vi "Netburner_cntl2.vi"() -> ()   [LabVIEW 2013]
panel:
  out "#  Bytes Read last":u32
  out "ADC last":string
  in  "Number of Cycles":i32=100
  out "ADC result":string
  out "#  Bytes Read":u32
  in  "ADC String  (Chan, #reads)":string="0 100"
  in  "2nd DAC String  (Chan, Volt)":string="1 -1."
  in  "1st DAC String  (Chan, Volt)":string="0 1"
  out "Error Out":errorcluster={"status"=FALSE, "code"=1073676294, "source"="VISA Read in Netburner_RD.vi->Netburner_cntl.vi"}
  in  "Error In (none)":errorcluster
  in  "COM Port #":refnum<visa-resource-name>="COM3"
  # "Netburner ADC/DAC Test Interface"
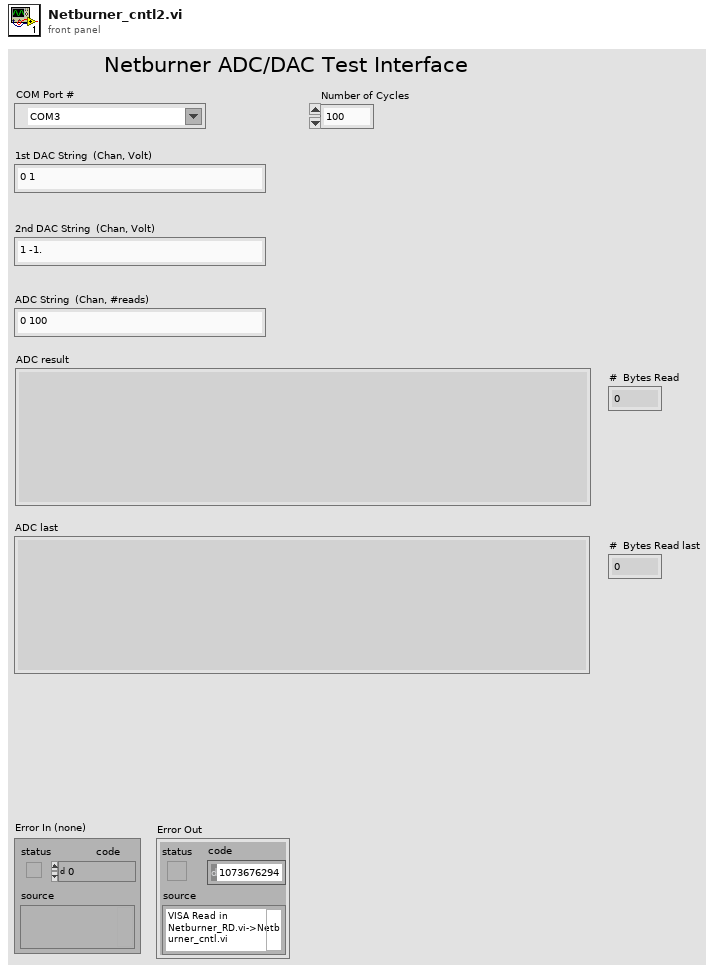
[diagram p1: front panel]
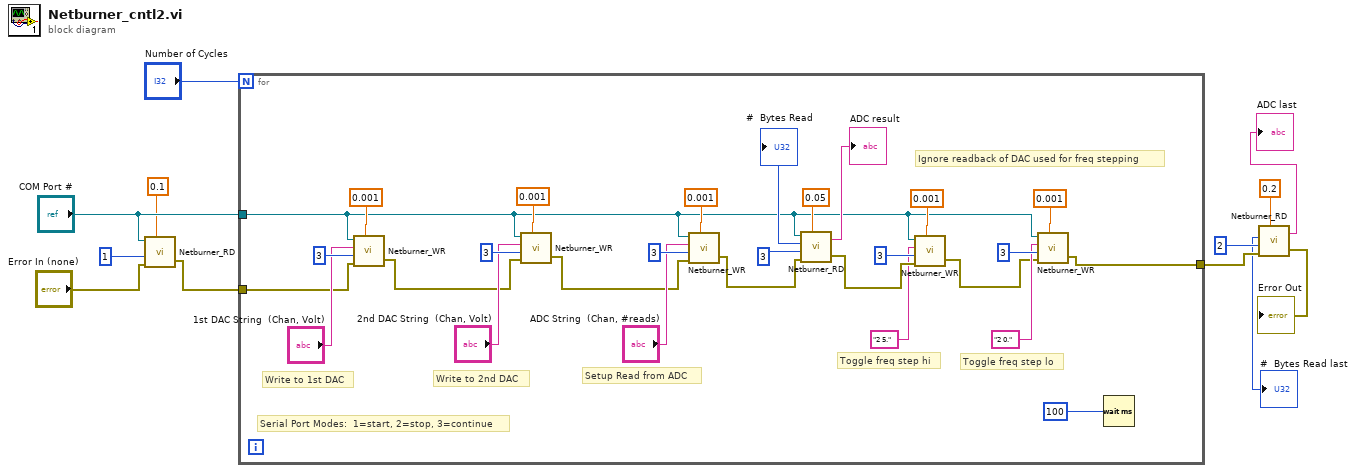
[diagram p0: block diagram]
diagram:
  n1 = call "Netburner_RD.vi"("VISA resource name (COM Port #)"="COM Port #", "Mode (0)"=1, "Error In (no error)"="Error In (none)", "Wait (sec)"=0.1) -> ("Error Out"=w10:errorcluster)  [unwired: 2 out]
  n2 = for {
    N: "Number of Cycles" -> [_]
    tunnel: "COM Port #" -> [w22]
    tunnel: w10 -> [w18]
    tunnel: [w14] -> w6
    # "Ignore readback of DAC used for freq stepping"
    # "Serial Port Modes:  1=start, 2=stop, 3=continue"
    # "Toggle freq step lo"
    # "Toggle freq step hi"
    # "Setup Read from ADC"
    # "Write to 2nd DAC"
    # "Write to 1st DAC"
    n3 = call "Netburner_WR.vi"("VISA resource name (COM Port #)"=w22, "String to Send"="1st DAC String  (Chan, Volt)", "Mode (0)"=3, "Error In (no error)"=w18, "Wait (sec)"=0.001) -> ("Error Out"=w17:errorcluster)  [unwired: 1 in]
    n4 = call "Netburner_WR.vi"("VISA resource name (COM Port #)"=w22, "String to Send"="2nd DAC String  (Chan, Volt)", "Mode (0)"=3, "Error In (no error)"=w17, "Wait (sec)"=0.001) -> ("Error Out"=w16:errorcluster)  [unwired: 1 in]
    n5 = call "Netburner_WR.vi"("VISA resource name (COM Port #)"=w22, "String to Send"="ADC String  (Chan, #reads)", "Mode (0)"=3, "Error In (no error)"=w16, "Wait (sec)"=0.001) -> ("Error Out"=w27:errorcluster)  [unwired: 1 in]
    n6 = call "Netburner_RD.vi"("VISA resource name (COM Port #)"=w22, "Mode (0)"=3, "Error In (no error)"=w27, "Wait (sec)"=0.05) -> ("Number of Bytes Received"=→"#  Bytes Read":u32, "Return String from Device"=→"ADC result":string, "Error Out"=w21:errorcluster)
    n7 = call "Netburner_WR.vi"("VISA resource name (COM Port #)"=w22, "String to Send"="2 5." ("1st DAC String to Send  (Channel, Voltage) 2"), "Mode (0)"=3, "Error In (no error)"=w21, "Wait (sec)"=0.001) -> ("Error Out"=w15:errorcluster)  [unwired: 1 in]
    n8 = call "Netburner_WR.vi"("VISA resource name (COM Port #)"=w22, "String to Send"="2 0." ("1st DAC String to Send  (Channel, Voltage) 2"), "Mode (0)"=3, "Error In (no error)"=w15, "Wait (sec)"=0.001) -> ("Error Out"=w14:errorcluster)  [unwired: 1 in]
    n9 = Wait (ms)(milliseconds to wait=100) -> ()  [unwired: 1 out]
  }
  n10 = call "Netburner_RD.vi"("Mode (0)"=2, "Error In (no error)"=w6, "Wait (sec)"=0.2) -> ("Number of Bytes Received"=→"#  Bytes Read last":u32, "Return String from Device"=→"ADC last":string, "Error Out"=→"Error Out":errorcluster)  [unwired: 1 in]
